vi "Deadband Filter.vi"(11 "Joystick axis":dbl) -> (3 "Filtered axis":dbl)   [LabVIEW 2017]
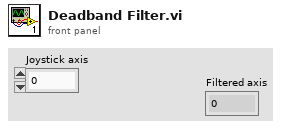
[diagram p1: front panel]
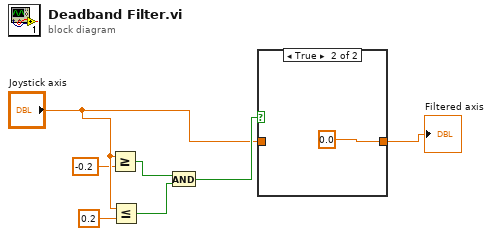
[diagram p0: block diagram]
diagram:
  n1 = Greater Or Equal?(x="Joystick axis", y=-0.2) -> (x >= y?=w1:bool)
  n2 = Less Or Equal?(x="Joystick axis", y=0.2) -> (x <= y?=w2:bool)
  n3 = And(x=w1, y=w2) -> (x .and. y?=w6:bool)
  n4 = case shown="True" w6 {
    tunnel: "Joystick axis" -> [w8 _]
    tunnel: [w8 0.0 ("Joystick axis")] -> w7
    frame False {
    }
    frame True {
    }
  }
  "Filtered axis" <- w7
